vi "ValveGUI.vi"() -> ()   [LabVIEW 2023, in "VolatusScratch.lvlib"]
uses:
  VolatusScratch.lvlib
  volatus-gui-controls/VolatusGUIControls/ImageButton.ctl
  volatus-gui-controls/VolatusGUIControls/VolatusGUIControls.lvlib
panel:
  out "avg_calc":cluster{"Color":u32, "Value":dbl}
  in  "avg_input":dbl(slide) scale=0.0..1000.0
  out "sum_calc":cluster{"Color":u32, "Value":dbl}
  in  "sum_b":dbl(slide) scale=0.0..1000.0
  in  "sum_a":dbl(slide) scale=0.0..10.0
  in  "GUI Link":bool
  in  "Group Logging Control":T1
  in  "Cycles_SP":T2 {"Value" format="%.3f"}
  out "BoolTest":bool
  in  "Done":T2
  in  "Remaining":T2
  out "Heat 3":bool
  in  "BluelinesRedlines":T3
  in  "DO10":cluster{"Picture":picture, "Command":bool}={"Picture"=bytes[9690], "Command"=FALSE}
  in  "DO09":cluster{"Picture":picture, "Command":bool}={"Picture"=bytes[9690], "Command"=FALSE}
  in  "DO08":cluster{"Picture":picture, "Command":bool}={"Picture"=bytes[9690], "Command"=FALSE}
  in  "DO04":cluster{"Picture":picture, "Command":bool}={"Picture"=bytes[9690], "Command"=FALSE}
  in  "ImageButton":T4={"Picture"=bytes[3230], "Button"=FALSE}
  out "Chart":cluster{"X":dbl[], "Y":dbl[]}[](graph)
  out "Cool 2":bool
  out "Heat 2":bool
  in  "Ox PSI":dbl(slide) scale=0.0..1000.0
  in  "Sequencing":T5={"Sequences"=[], "Unload All"=FALSE, "Abort All"=FALSE, "Loaded, Good CRC"=13816530, "Sequence Error"=16744319, "Loaded, CRC Mismatch"=16777142, "Running, Good CRC"=11730866, "Unloaded"=7171459, "Running, CRC Mismatch"=10530559}
  out "Cool":bool
  out "Heat":bool
  in  "Fuel PSI":dbl(slide) scale=0.0..1000.0
  out "BB PV":cluster{"Color":u32, "Value":dbl}
  in  "Fill":cluster{"Color":u32, "Button":bool}
  in  "Low High":T2
  in  "Low Low":T2
  in  "Mid High":T2
  in  "Mid Low":T2
  in  "High High":T2
  in  "High Low":T2
  in  "BangBang":cluster{"Color":u32, "Button":bool}
  in  "Fill Lower":T2
  in  "Fill Upper":T2
  in  "Ox_Level_3":dbl(slide) scale=0.0..400.0
  in  "Ox_Level_2":dbl(slide) scale=0.0..400.0
  in  "Ox_Level_1":dbl(slide) scale=0.0..400.0
  in  "Ox_PT_03":dbl(slide) scale=0.0..1000.0
  in  "Ox_PT_02":dbl(slide) scale=0.0..1000.0
  in  "Ox_PT_01":dbl(slide) scale=0.0..1000.0
  in  "Low":cluster{"Picture":picture, "Command":bool}={"Picture"=bytes[9690], "Command"=FALSE}
  in  "Mid":cluster{"Picture":picture, "Command":bool}={"Picture"=bytes[9690], "Command"=FALSE}
  in  "High":cluster{"Picture":picture, "Command":bool}={"Picture"=bytes[9690], "Command"=FALSE}
  in  "Logging Control":T6
  in  "System Config Status":T7
  # "Low"
  # "Value"
  # "High"
  # "Low"
  # "Value"
  # "High"
  # "Sequence"
  # "State"
  # "State Time"
  # "Seq Time"
  # "Started"
  # "Config Status"
  # "Ver"
  # "Hash"
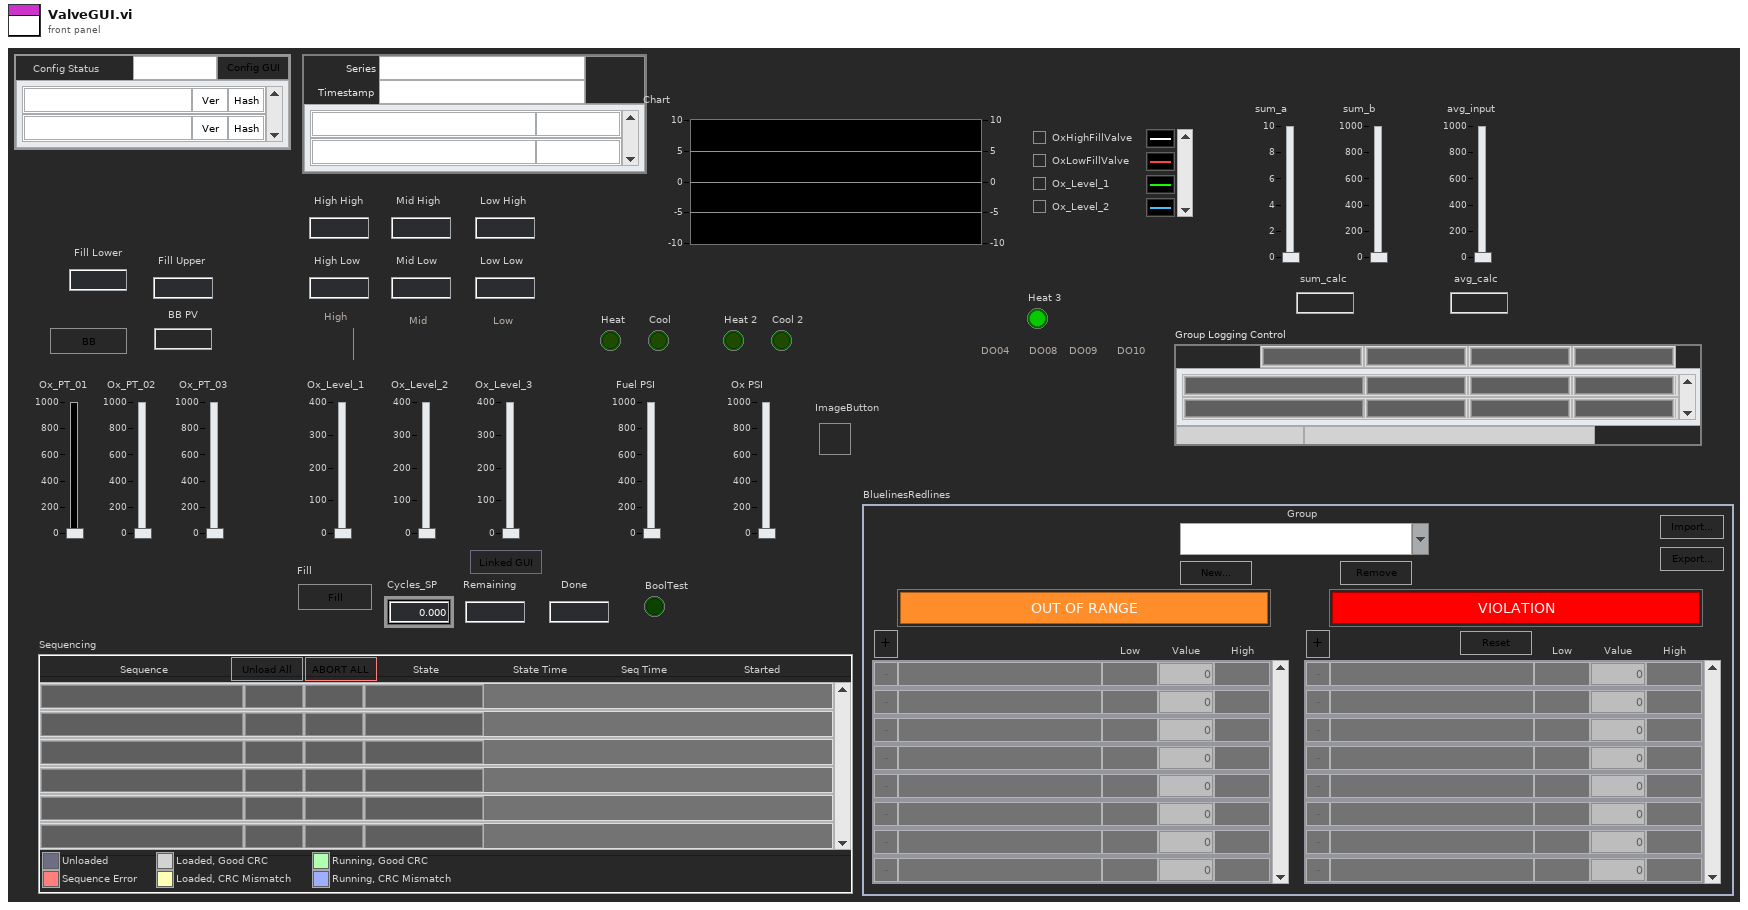
[diagram p1: front panel]
types:
  T1 = cluster{"Series":string, "Timestamp":string, "Targets":cluster{"Node":string, "Node Color":u32, "Groups":cluster{"Group":string, "Group Color":u32, "Button":bool}[]}[], "Groups":cluster{"Group":string, "Group Color":u32, "Button":bool}[]}
  T2 = cluster{"Color":u32, "Value":dbl, "Backdrop":bool}
  T3 = cluster{"Blue Lines":cluster{"Channel":string, "Low":string, "Value":dbl, "High":string, "Color":u32, "Remove Channel":bool}[], "Red Lines":cluster{"Channel":string, "Low":string, "Value":dbl, "High":string, "Color":u32, "Remove Channel":bool}[], "Import":bool, "Export":bool, "Blueline Status":bool, "Redlines Status":bool, "Group":string, "New Group":bool, "Dup Group":bool, "Remove Group":bool, "Add Blue Channel":bool, "Add Red Channel":bool, "Reset Redlines":bool}
  T4 = typedef "VolatusGUIControls.lvlib/ImageButton.ctl" = cluster{"Picture":picture, "Button":bool}
  T5 = cluster{"Sequences":cluster{"Name Color":u32, "Name":string, "Btn 1 Color":u32, "Btn 1 Text":string, "Btn 2 Color":u32, "Btn 2 Text":string, "Status Color":u32, "Status":string, "State Time":string, "Started":string, "Seq Time":string, "Btn 1":bool, "Btn 2":bool, "Btn Name":bool}[], "Unload All":bool, "Abort All":bool, "Loaded, Good CRC":u32, "Sequence Error":u32, "Loaded, CRC Mismatch":u32, "Running, Good CRC":u32, "Unloaded":u32, "Running, CRC Mismatch":u32}
  T6 = cluster{"Series":string, "Timestamp":string, "Log Button":bool, "Status":cluster{"Node":string, "Node Color":u32, "State":string}[]}
  T7 = cluster{"Status Color":u32, "Status String":string, "Config GUI":bool, "Status":cluster{"Node Name":string, "Node Color":u32, "Version Color":u32, "Hash Color":u32}[]}
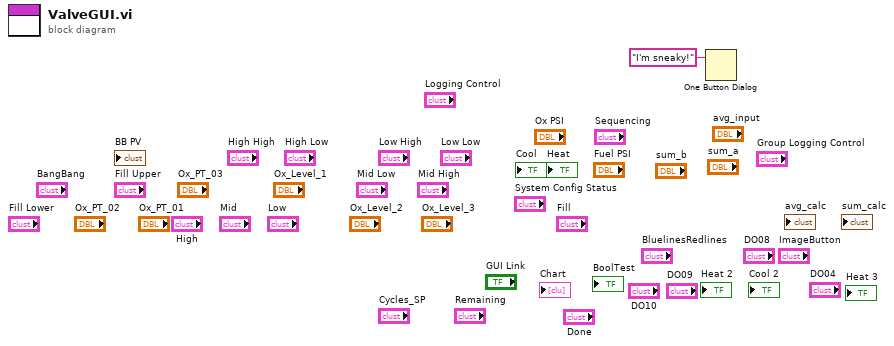
[diagram p0: block diagram]
diagram:
  n1 = One Button Dialog(message="I'm sneaky!") -> ()  [unwired: 1 in, 1 out]
